vi "Format Parameter String from Cluster.vi"(8 "error in (no error)":errorcluster, 11 "Variant":variant) -> (0 "error out":errorcluster, 3 "String":string)   [LabVIEW 2010]
doc: "Creates a formated text string of parameter Name - Value pairs from a variant of an input cluster.\n\nThe string is of the format: name1=value1, ... nameN=valueN"
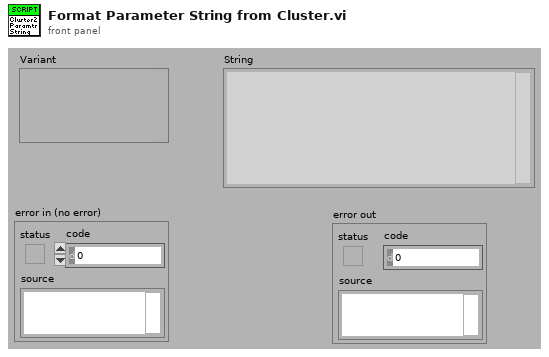
[diagram p1: front panel]
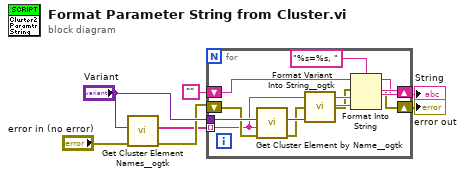
[diagram p0: block diagram]
diagram:
  n1 = call <userlib>:"Get Cluster Element Names__ogtk.vi"("error in (no error)"="error in (no error)", "Cluster"="Variant") -> ("error out"=w5:errorcluster, "Element Names"=w3:string[])  [unwired: 8 in]
  n2 = for {
    tunnel: "Variant" -> [w18]
    tunnel: w3 -> [w12] mode=indexing
    shift-right: [w13] -> w1
    shift-left: "" -> [w14]
    shift-right: [w9] -> w2
    shift-left: w5 -> [w15]
    n3 = call <userlib>:"Get Cluster Element by Name__ogtk.vi"("error in (no error)"=w15, "Element Name"=w12, "Cluster"=w18) -> ("error out"=w16:errorcluster, "VElement"=w17:variant)  [unwired: 6 in, 1 out]
    n4 = call <userlib>:"Format Variant Into String__ogtk.vi"("error in (no error)"=w16, "Variant"=w17) -> ("Output String"=w11:string, "error out"=w10:errorcluster)  [unwired: 12 in]
    n5 = Format Into String(format string="%s=%s, ", initial string=w14, error in=w10, w12, w11) -> (resulting string=w13:string, error out=w9:errorcluster)
  }
  "error out" <- w2
  "String" <- w1
